vi "Channel Setting_2.vi"(8 "에러 입력(에러 없음)":errorcluster, 11 "Device Item Ref in":T1 format="%.0x") -> (0 "에러 출력":errorcluster, 3 "Parent Ref out":T1 format="%.0x")   [LabVIEW 2017, in "Serial Communcation Devices Custom Device.lvlib"]
uses:
  Serial Communcation Devices Custom Device.lvlib
  <vilib>/NI Veristand/Custom Device API/Custom Device Channel Type.ctl
  <vilib>/NI Veristand/Custom Device API/Custom Device API.lvlib
  <vilib>/NI Veristand/Custom Device API/Custom Device Item Ref.ctl
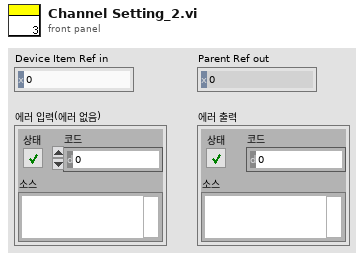
[diagram p1: front panel]
types:
  T1 = typedef "Custom Device API.lvlib/Custom Device Item Ref.ctl" = u64
  T2 = typedef "Custom Device API.lvlib/Custom Device Channel Type.ctl" = enum16{"Input", "Output"}
  T3 = cluster{"Type":T2, "Units":string, "Default Value":dbl, "Faultable":bool, "Scalable":bool}
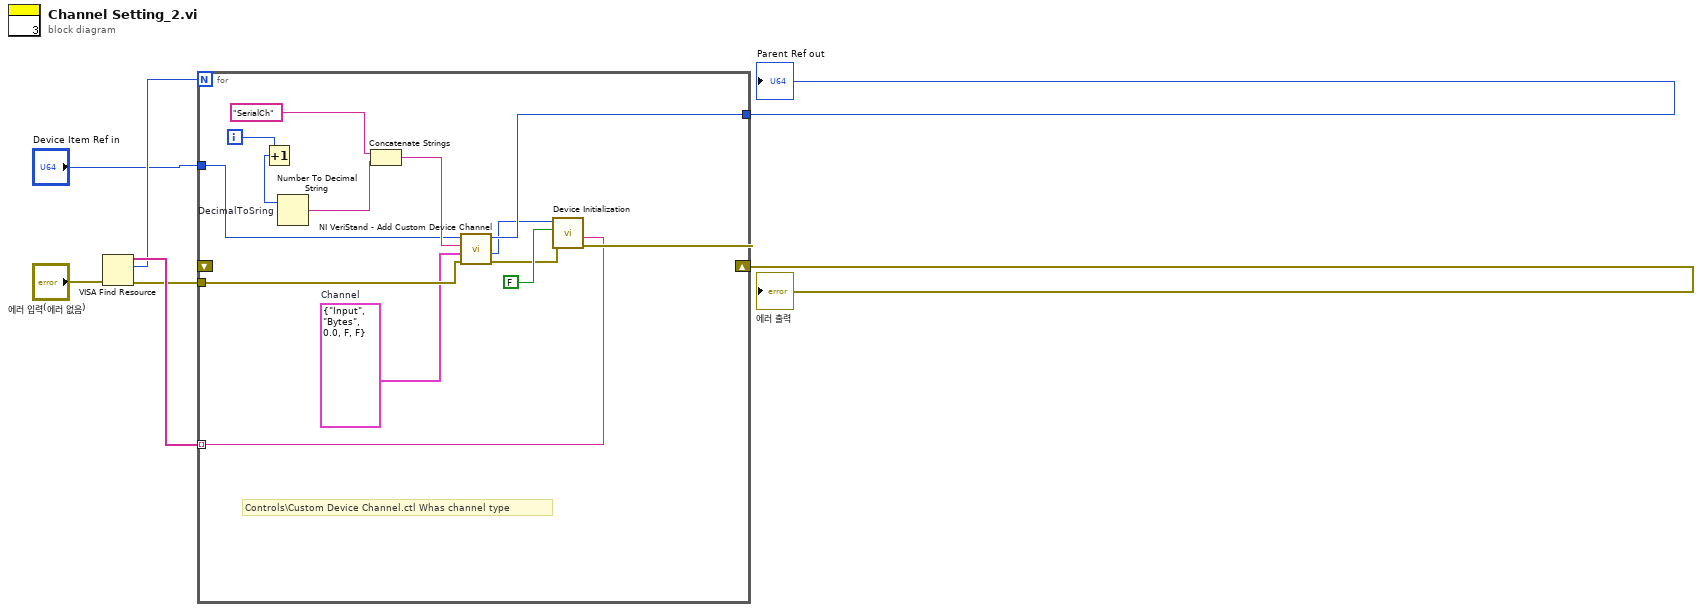
[diagram p0: block diagram]
diagram:
  n1 = VISA Find Resource(8:"에러 입력(에러 없음)") -> (0:w6:errorcluster, 2:w4:u32, 3:w7:string[])  [unwired: 2 in]
  n2 = for {
    N: w4 -> [_]
    tunnel: w6 -> [w19]
    tunnel: "Device Item Ref in" -> [w16]
    tunnel: [w10] -> w3
    shift-right: [w11] -> w2
    shift-left: _ -> [_]
    tunnel: w7 -> [w8] mode=indexing
    i -> [w18]
    w12 = T3 {"Type"=enum."Input", "Units"="Bytes", "Default Value"=0.0, "Faultable"=FALSE, "Scalable"=FALSE}  # Channel
    # "Controls\\Custom Device Channel.ctl Whas channel type"
    n3 = Increment(x=w18) -> (x+1=w13:i32)
    n4 = Number To Decimal String "DecimalToSring"(number=w13) -> (decimal integer string=w14:string)  [unwired: 1 in]
    n5 = Concatenate Strings("SerialCh", w14) -> (w17:string)
    n6 = call <vilib>:"NI VeriStand - Add Custom Device Channel.vi"("error in (no error)"=w19, "Channel"=w12, "Channel Name"=w17, "Parent Ref in"=w16) -> ("error out"=w20:errorcluster, "Channel Ref"=w9:T1, "Parent Ref out"=w10:T1)  [unwired: 4 in, 1 out]
    n7 = call "Device Initialization.vi"("에러 입력(에러 없음)"=w20, "VISA Resource Name"=w8, 10:FALSE, "Channel Ref"=w9) -> ("에러 출력"=w11:errorcluster)  [unwired: 7 in]
  }
  "Parent Ref out" <- w3
  "에러 출력" <- w2
